vi "LJLogM.vi"() -> ()   [LabVIEW 2022 SP3]
panel:
  in  "Tab Control":enum32{"Original UI", "Page 2"}(tab)
  out "Error Message":string="No Error"
  in  "Write To File":bool
  in  "Data File Prefix":string="data"
  out "Current Data File":path=path "None"
  in  "Interval (ms)":u32=500
  out "# of iterations":i32
  in  "Name":string[](array[string])=["AIN0", "AIN1", "AIN2", "AIN3", "AIN4", "AIN5", "AIN6", "AIN7", "AIN8", "AIN9", "AIN10", "AIN11", "AIN12", "AIN13", "AIN14", "AIN15"]
  out "Value":dbl[](array[numeric]) format="%.6f"
  in  "# Channels":i32=4 min=1 max=16
  in  "Scaling Equation":string[](array[string])=["y=a", "y=b", "y=c", "y=d", "y=e", "y=f", "y=g", "y=h", "y=i", "y=j", "y=k", "y=l", "y=m", "y=n", "y=o", "y=p"]
  out "Scaled":dbl[](array[numeric]) format="%.6f"
  in  "exit":bool
  in  "# Scans On Graph":i32=1000 min=0
  out "Waveform Graph":cluster{dbl, dbl, dbl[][]}(graph)={0.0, 0.5, []}
  in  "Graph?":bool[](array[boolean])=[TRUE, FALSE, FALSE, FALSE, FALSE, FALSE, FALSE, FALSE, FALSE, FALSE, FALSE, FALSE, FALSE, FALSE, FALSE, FALSE]
  in  "Max File Size (Bytes)":i32=1048576 min=1 max=2000000000
  in  "Change Working Directory":bool
  out "DevType":i32
  out "ConnType":i32
  out "SerialNumber":i32
  out "ms per iteration":i32
  in  "Save Configuration":bool
  out "Device Config File Name":string="LJLogM.cfg"
  # "0"
  # "1"
  # "2"
  # "3"
  # "Original UI, don't edit\nunless you're sure of \nwhat you're doing"
  # "4"
  # "5"
  # "6"
  # "7"
  # "8"
  # "9"
  # "10"
  # "11"
  # "12"
  # "13"
  # "14"
  # "15"
  # "- \"a\" - \"p\" correspond to the raw Voltage value from the \n  1st through 16th row.\n- The scaled output value is \"y\".\n- If your equation has an error, the output will be zero."
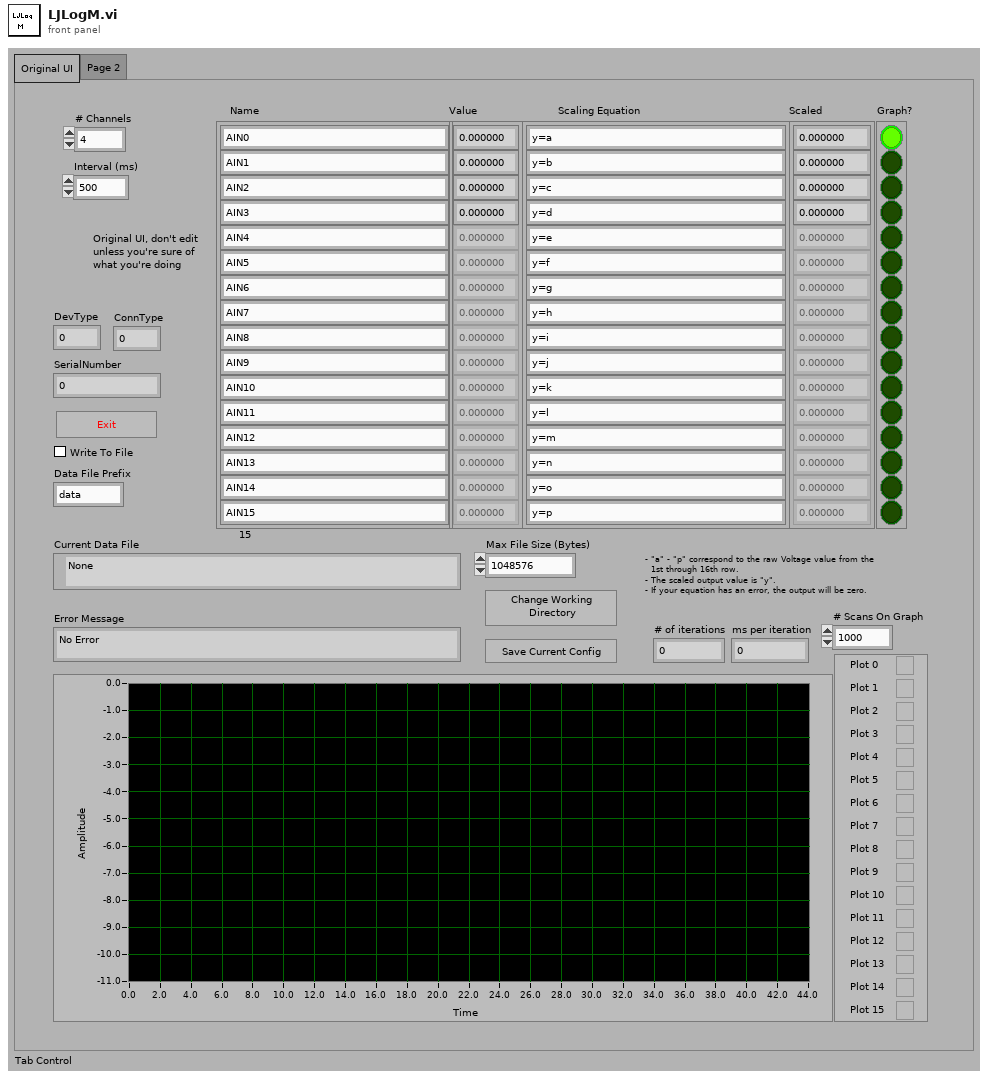
[diagram p1: front panel]
types:
  T1 = cluster{"+Ch":string[], "-Ch":string[], "Ranges":u16[], "Scaling Equation":string[], "Graph?":bool[]}
  T2 = cluster{"# Channels":i32, "Name":string[], string[], u16[], "Scaling Equation":string[]}
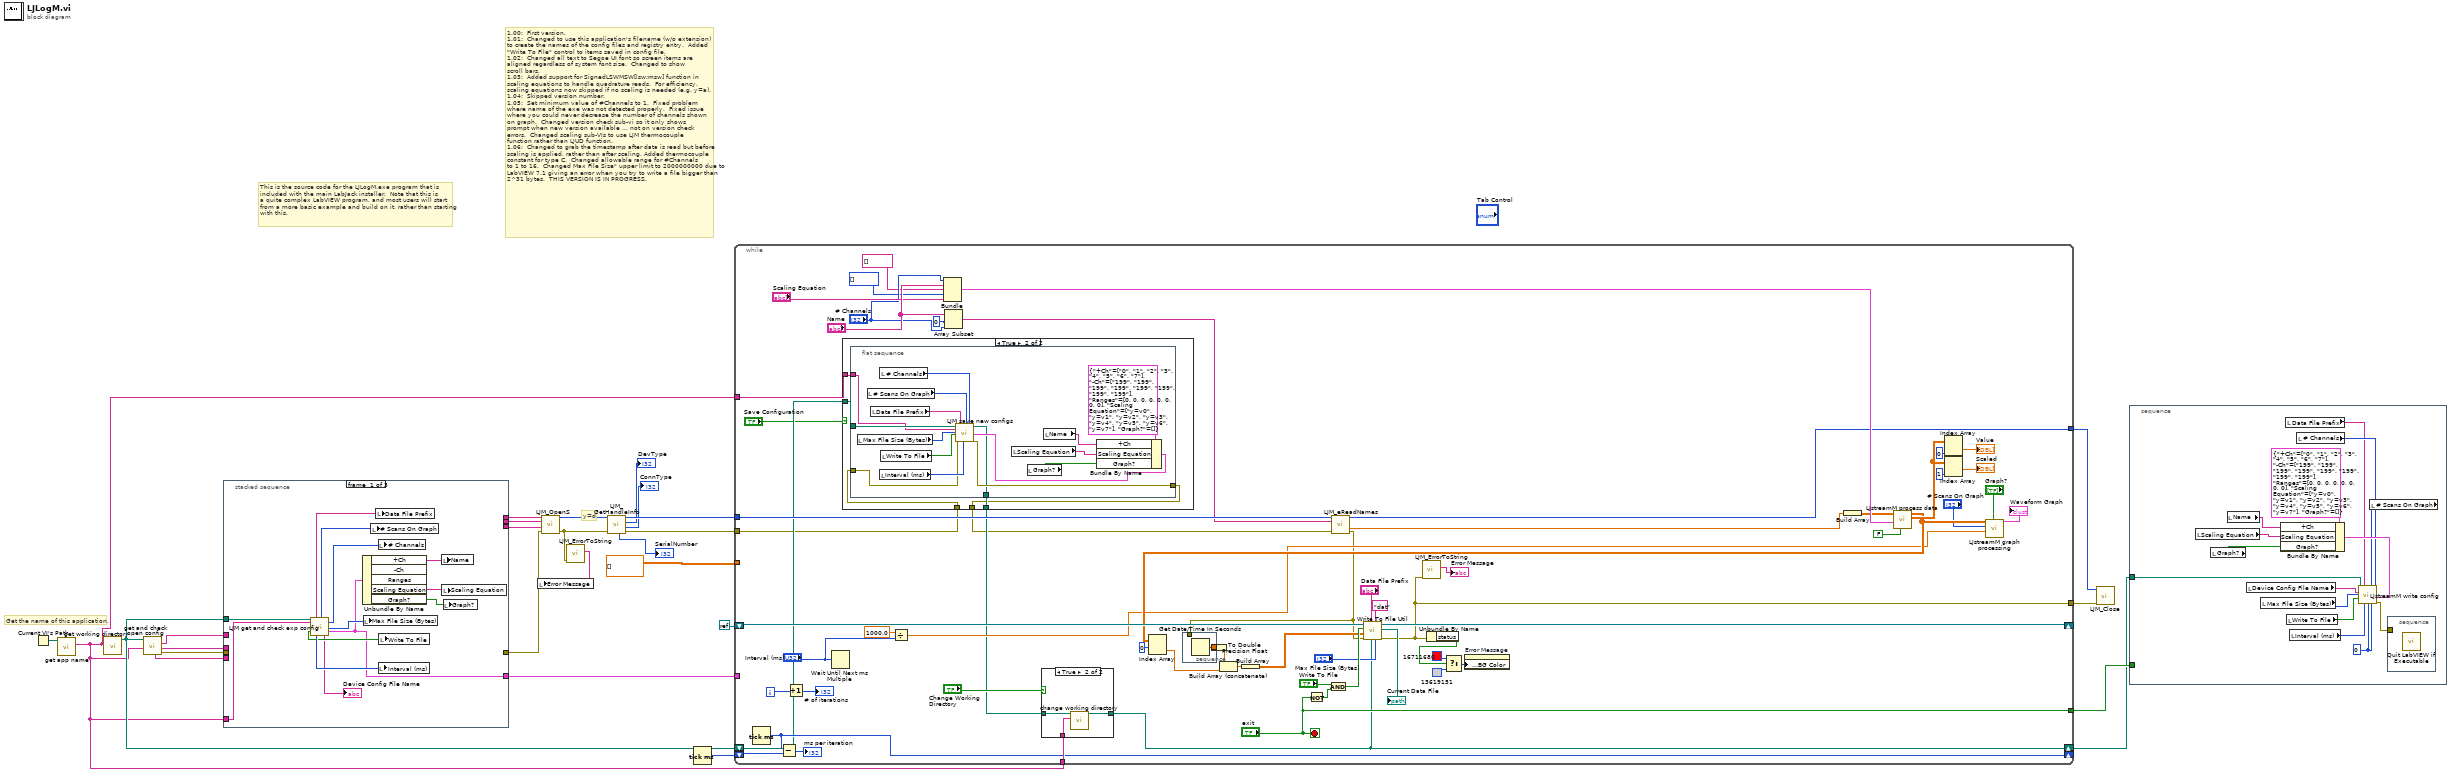
[diagram p0: block diagram]
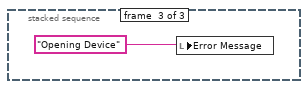
[diagram p5: hidden frame]
diagram:
  # "y=d"
  # "This is the source code for the LJLogM.exe program that is\nincluded with the main LabJack installer.  Note that this is \na quite complex LabVIEW program, and most users will start\nfrom a more basic example and build on it, rather than starting\nwith this."
  # "Get the name of this application."
  # "1.00:  First version.\n1.01:  Changed to use this application's filename (w/o extension)\nto create the names of the config files and registry entry.  Added\n\"Write To File\" control to items saved in config file.\n1.02:  Changed all text to Segoe UI font so screen items are\naligned regardless of system font size.  Changed to show\nscroll bars.\n1.03:  Added support for SignedLSWMSW[lsw:msw] function in\nscaling equations to handle quadrature reads.  For efficiency,\nscaling equations now skipped if no scaling is needed (e.g. y=a).\n1.04:  Skipped version number.\n1.05:  Set minimum value of #Channels to 1.  Fixed problem\nwhere name of the exe was not detected properly.  Fixed issue\nwhere you could never decrease the number of channels shown\non graph.  Changed version check sub-vi so it only shows\nprompt when new version available ... not on version check\nerrors.  Changed scaling sub-VIs to use LJM thermocouple\nfunction rather than LJUD function.\n1.06:  Changed to grab the timestamp after data is read but before\nscaling is applied, rather than after scaling. Added thermocouple\nconstant for type C.  Changed allowable range for #Channels\nto 1 to 16.  Changed Max File Size\" upper limit to 2000000000 due to\nLabVIEW 7.1 giving an error when you try to write a file bigger than\n2^31 bytes.  THIS VERSION IS IN PROGRESS."
  n1 = Current VI's Path() -> (path=w9:path)
  n2 = call "get app name.vi"("Current VI's Path"=w9) -> ("App Name Without Extension"=w1:string)  [unwired: 4 in, 2 out]
  n3 = call "get working directory.vi"("Application Name"=w1) -> ("Working Directory"=w2:path)  [unwired: 9 in, 1 out]
  n4 = call "get and check open config.vi"("App Name"=w1, "Working Directory In"=w2) -> ("error out"=w4:errorcluster, "ConnectionType"=w6:string, "DeviceType"=w7:string, "Identifier"=w5:string)  [unwired: 4 in, 2 out]
  n5 = stacked-sequence {
    tunnel: [w29 _ _] -> w25
    tunnel: [_ w44 _] -> w17
    tunnel: [_ w43 _] -> w16
    tunnel: [_ w42 _] -> w15
    tunnel: w7 -> [_ w44 _]
    tunnel: w6 -> [_ w43 _]
    tunnel: w5 -> [_ w42 _]
    tunnel: w4 -> [_ w41 _]
    tunnel: [_ w41 _] -> w3
    tunnel: w2 -> [w32 _ _]
    tunnel: w1 -> [w31 _ _]
    frame #0 {
      n6 = call "LJM get and check exp config.vi"("Working Directory In"=w32, "App Name"=w31) -> ("Write To File"=w36:bool, "Data File Prefix"=w33:string, "Interval (ms)"=w37:u32, "Graph History"=w34:i32, "Device Config File Name"=→"Device Config File Name":string, "# Channels"=w28:i32, "Max File Size (Bytes)"=w35:i32, "Channel Setup"=w29:T1)  [unwired: 6 in, 4 out]
      n7 = Unbundle By Name(w29) -> ("+Ch"=w39:string[], "Scaling Equation"=w40:string[], "Graph?"=w38:bool[])  [unwired: 2 out]
      n8 = local write "Max File Size (Bytes)"(w35) -> ()
      n9 = local write "# Scans On Graph"(w34) -> ()
      n10 = local write "Data File Prefix"(w33) -> ()
      n11 = local write "# Channels"(w28) -> ()
      n12 = local write "Interval (ms)"(w37) -> ()
      n13 = local write "Write To File"(w36) -> ()
      n14 = local write "Name"(w39) -> ()
      n15 = local write "Scaling Equation"(w40) -> ()
      n16 = local write "Graph?"(w38) -> ()
    }
    frame #1 {
    }
    frame #2 {
      n17 = local write "Error Message"("Opening Device" ("Error Message")) -> ()
    }
  }
  n18 = call "LJM_OpenS.vi"("error in"=w3, "Identifier"=w15, "ConnectionType"=w16, "DeviceType"=w17) -> ("error out"=w14:errorcluster, "Handle"=w21:i32)  [unwired: 6 in]
  n19 = call "LJM_ErrorToString.vi"("error in"=w14) -> ("String"=w13:string)  [unwired: 10 in]
  n20 = local write "Error Message"(w13) -> ()
  n21 = call "LJM_GetHandleInfo.vi"("error in"=w14, "Handle In"=w21) -> ("error out"=w23:errorcluster, "ConnectionType"=→"ConnType":i32, "DeviceType"=→"DevType":i32, "Handle Out"=w22:i32, "SerialNumber"=→"SerialNumber":i32)  [unwired: 2 in, 3 out]
  n22 = Tick Count (ms)() -> (millisecond timer value=w10:u32)
  n23 = while {
    shift-left: w2 -> [w51]
    shift-right: [w64] -> w8
    tunnel: w1 -> [w65]
    tunnel: dbl[][] [] ("Waveform Chart") -> [_]
    tunnel: w23 -> [w49]
    tunnel: w22 -> [w63]
    shift-left: refnum<k0> refnum -> [w93]
    shift-right: [w95] -> _
    tunnel: w25 -> [_]
    tunnel: ["exit"] -> w24
    tunnel: [w57] -> w12
    tunnel: [w56] -> w11
    shift-right: [w53] -> _
    shift-left: w10 -> [w55]
    tunnel: w1 -> [w46]
    i -> [w100]
    stop <- "exit" stop-if-true
    n24 = Tick Count (ms)() -> (millisecond timer value=w53:u32)
    n25 = Subtract(x=w53, y=w55) -> (x-y=→"ms per iteration":u32)
    n26 = Increment(x=w100) -> (x+1=→"# of iterations":i32)
    n27 = Wait Until Next ms Multiple(millisecond multiple="Interval (ms)") -> ()  [unwired: 1 out]
    n28 = case shown="True" "Save Configuration" {
      tunnel: w51 -> [w108 w113]
      tunnel: [w108 w112] -> w50
      tunnel: w49 -> [w107 w111]
      tunnel: [w107 w110] -> w48
      tunnel: w46 -> [_ w109]
      frame False {
      }
      frame True {
        n29 = flat-sequence {
          tunnel: w113 -> [w126]
          tunnel: [w116] -> w112
          tunnel: w111 -> [w120]
          tunnel: [w119] -> w110
          tunnel: w109 -> [w114]
          frame #0 {
            n30 = local read "Max File Size (Bytes)"() -> (w117:i32)
            n31 = local read "# Scans On Graph"() -> (w129:i32)
            n32 = local read "Data File Prefix"() -> (w115:string)
            n33 = local read "Interval (ms)"() -> (w127:u32)
            n34 = local read "# Channels"() -> (w128:i32)
            n35 = local read "Write To File"() -> (w118:bool)
            n36 = local read "Scaling Equation"() -> (w124:string[])
            n37 = local read "Graph?"() -> (w125:bool[])
            n38 = local read "Name"() -> (w123:string[])
            n39 = Bundle By Name(cluster=T1 {"+Ch"=["0", "1", "2", "3", "4", "5", "6", "7"], "-Ch"=["199", "199", "199", "199", "199", "199", "199", "199"], "Ranges"=[0, 0, 0, 0, 0, 0, 0, 0], "Scaling Equation"=["y=v0", "y=v1", "y=v2", "y=v3", "y=v4", "y=v5", "y=v6", "y=v7"], "Graph?"=[]} ("Channel Setup"), "+Ch"=w123, "Scaling Equation"=w124, "Graph?"=w125) -> (w121:T1)
            n40 = call "LJM save new configs.vi"("Working Directory"=w126, "App name"=w114, "Max File Size (Bytes)"=w117, "Write To File"=w118, "error in"=w120, "Data File Prefix"=w115, "Interval (ms)"=w127, "Graph History"=w129, "# Channels"=w128, "Channel Setup"=w121) -> ("Working Directory Out"=w116:path, "error out"=w119:errorcluster)  [unwired: 8 in]
          }
        }
      }
    }
    n41 = Divide(x=1000.0, y="Interval (ms)") -> (x/y=w73:dbl)
    n42 = Bundle("# Channels"="# Channels", "Name"="Name", string[] [], u16[] [], "Scaling Equation"="Scaling Equation") -> (w90:T2)  [unwired: 1 in]
    n43 = Array Subset(array="Name", index=0 ("Array Index"), length="# Channels") -> (w62:string[])
    n44 = case shown="True" "Change Working Directory" {
      tunnel: w65 -> [_ w131]
      tunnel: w50 -> [w130 w133]
      tunnel: [w130 w132] -> w64
      frame False {
      }
      frame True {
        n45 = call "change working directory.vi"("Application Name"=w131, "Working Directory In"=w133) -> ("Working Directory Out"=w132:path)  [unwired: 9 in]
      }
    }
    n46 = Not(x="exit") -> (.not. x?=w102:bool)
    n47 = And(x="Write To File", y=w102) -> (x .and. y?=w94:bool)
    n48 = call "LJM_eReadNames.vi"("Handle In"=w63, "aNames"=w62, "error in"=w48) -> ("Handle Out"=w56:i32, "aValuesOut"=w58:dbl[], "error out"=w52:errorcluster)  [unwired: 9 in, 1 out]
    n49 = stacked-sequence {
      tunnel: [w135] -> w87
      tunnel: w52 -> [_]
      frame #0 {
        n50 = Get Date/Time In Seconds() -> (seconds since 1Jan1904=w134:timestamp)
        n51 = To Double Precision Float(number=w134) -> (double precision float=w135:dbl)
      }
    }
    n52 = Build Array(w58) -> (w85:dbl[][])
    n53 = call "LJstreamM process data.vi"("Disable Scaling"=FALSE, "Channel Config"=w90, "Voltages"=w85) -> ("Volts,Scaled Averages"=w89:dbl[][], "Scaled Data"=w78:dbl[][])  [unwired: 7 in]
    n54 = Index Array(array=w78, index (row)=0 ("Index (row)")) -> (element=w83:dbl[])  [unwired: 1 in]
    n55 = Build Array (concatenate)(w87, w83) -> (w86:dbl[])
    n56 = Build Array(w86) -> (w82:dbl[][])
    n57 = call "Write To File Util.vi"("Maximum File Size (Bytes)"="Max File Size (Bytes)", "Data File Extension"="dat", "Working Directory"=w64, "Data File Prefix"="Data File Prefix", "error in"=w52, "Data"=w82, "Write To File"=w94, "File Refnum In"=w93) -> ("error out"=w57:errorcluster, "Current Data File"=→"Current Data File":path, "File Refnum Out"=w95:refnum<file>)  [unwired: 1 in]
    n58 = call "LJM_ErrorToString.vi"("error in"=w57) -> ("String"=→"Error Message":string)  [unwired: 10 in]
    n59 = Unbundle By Name(w57) -> ("status"=w70:bool)
    n60 = Select(t=u32 16711680, s=w70, f=u32 13619151) -> (s? t:f=w69:u32)
    n61 = property on="Error Message" class="Str"("Text.Text Colors:BG Color"=w69) -> ()  [unwired: 2 in, 2 out]
    n62 = Index Array(array=w89, index (col)=0 ("Disabled Index (col)")) -> (element=→"Value":dbl[])  [unwired: 1 in]
    n63 = Index Array(array=w89, index (col)=1 ("Disabled Index (col)")) -> (element=→"Scaled":dbl[])  [unwired: 1 in]
    n64 = call "LJstreamM graph processing.vi"("Graph?"="Graph?", "Scan Rate"=w73, "Graph History (# scans)"="# Scans On Graph", "Scaled Data"=w78) -> ("Graph Data"=→"Waveform Graph":cluster{dbl, dbl, dbl[][]})  [unwired: 7 in]
  }
  n65 = call "LJM_Close.vi"("error in"=w12, "Handle"=w11) -> ()  [unwired: 9 in, 1 out]
  n66 = stacked-sequence {
    tunnel: w8 -> [w136]
    tunnel: w24 -> [_]
    frame #0 {
      w145 = u8 0 ("Resolution")
      n67 = local read "Scaling Equation"() -> (w148:string[])
      n68 = local read "Graph?"() -> (w147:bool[])
      n69 = local read "Name"() -> (w149:string[])
      n70 = local read "Device Config File Name"() -> (w137:string)
      n71 = local read "Max File Size (Bytes)"() -> (w139:i32)
      n72 = Bundle By Name(cluster=T1 {"+Ch"=["0", "1", "2", "3", "4", "5", "6", "7"], "-Ch"=["199", "199", "199", "199", "199", "199", "199", "199"], "Ranges"=[0, 0, 0, 0, 0, 0, 0, 0], "Scaling Equation"=["y=v0", "y=v1", "y=v2", "y=v3", "y=v4", "y=v5", "y=v6", "y=v7"], "Graph?"=[]} ("Channel Setup"), "+Ch"=w149, "Scaling Equation"=w148, "Graph?"=w147) -> (w143:T1)
      n73 = local read "Data File Prefix"() -> (w140:string)
      n74 = local read "Write To File"() -> (w138:bool)
      n75 = local read "Interval (ms)"() -> (w146:u32)
      n76 = local read "# Channels"() -> (w142:i32)
      n77 = local read "# Scans On Graph"() -> (w141:i32)
      n78 = call "LJstreamM write config.vi"("Working Directory"=w136, "Data File Prefix"=w140, "Graph History"=w141, "# Channels"=w142, "filename"=w137, "Max File Size (Bytes)"=w139, "Write To File"=w138, "Channel Setup"=w143, "Interval (ms)"=w146, "Resolution"=w145, "SettlingFactor"=w145) -> ("error out"=w144:errorcluster)  [unwired: 4 in]
      n79 = stacked-sequence {
        tunnel: w144 -> [_]
        frame #0 {
          n80 = call "Quit LabVIEW if Executable.vi"() -> ()  [unwired: 1 in]
        }
      }
    }
  }
